vi "Handle Messages_Template.vi"(8 "error in (no error)":errorcluster, 9 "Message Data":variant, 10 "Message":string, 11 "TRIARC_PROCESS_IN":refnum<class>) -> (0 "error out":errorcluster, 3 "TRIARC_PROCESS_OUT":refnum<class>)   [LabVIEW 2020]
uses:
  My Process 0/My Process 0ads.lvclass
  C:/Users/anton/Documents/GitHub/Triarc-Framework/source/Framework/Application/Application.lvclass
  C:/Users/anton/Documents/GitHub/Triarc-Framework/source/Framework/Process/Process.lvclass
  C:/Users/anton/Documents/GitHub/Triarc-Framework/source/Framework/Base/Base.lvclass
  C:/Users/anton/Documents/GitHub/Triarc-Framework/source/Framework/Configuration File/Configuration File.lvclass
  C:/Users/anton/Documents/GitHub/Triarc-Framework/source/My Process 0/My Process 0ads.lvclass
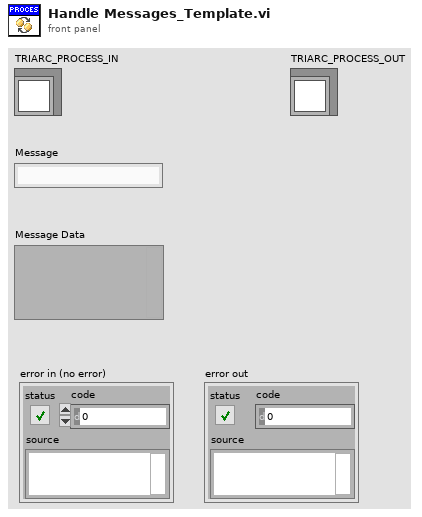
[diagram p1: front panel]
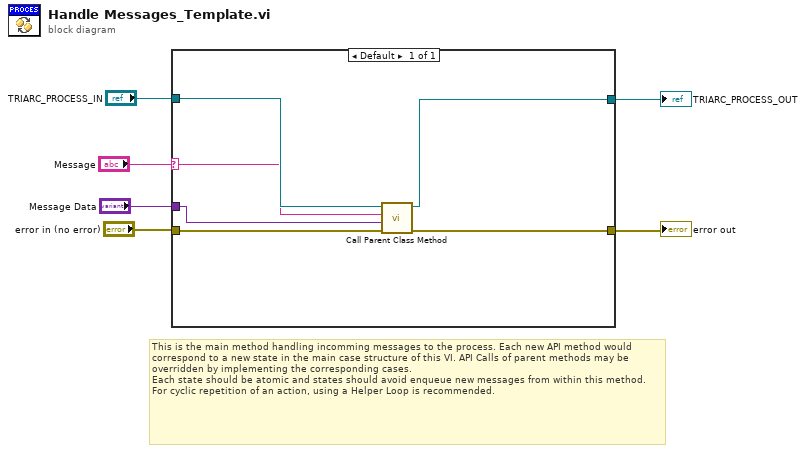
[diagram p0: block diagram]
diagram:
  # "This is the main method handling incomming messages to the process. Each new API method would correspond to a new state in the main case structure of this VI. API Calls of parent methods may be overridden by implementing the corresponding cases.\nEach state should be atomic and states should avoid enqueue new messages from within this method. For cyclic repetition of an action, using a Helper Loop is recommended."
  n1 = case shown="Default" "Message" {
    selector: "Message" -> [w10]
    tunnel: "error in (no error)" -> [w9]
    tunnel: "TRIARC_PROCESS_IN" -> [w12]
    tunnel: "Message Data" -> [w11]
    tunnel: [w8] -> w2
    tunnel: [w7] -> w1
    frame Default {
      n2 = call-parent "Call Parent Class Method"("error in (no error)"=w9, "Message Data"=w11, "Message"=w10, "Application In"=w12) -> ("error out"=w8:errorcluster, "Application Out"=w7:refnum<class "My Process 0ads.lvclass">)  [unwired: 6 in]
    }
  }
  "error out" <- w2
  "TRIARC_PROCESS_OUT" <- w1
